vi "Pulse Stretch & Delay.vi"(1 "Delay (sec)":dbl, 2 "In":bool, 4 "Width (sec)":dbl=0.01) -> (5 "Out":bool)   [LabVIEW 2013]
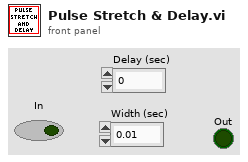
[diagram p1: front panel]
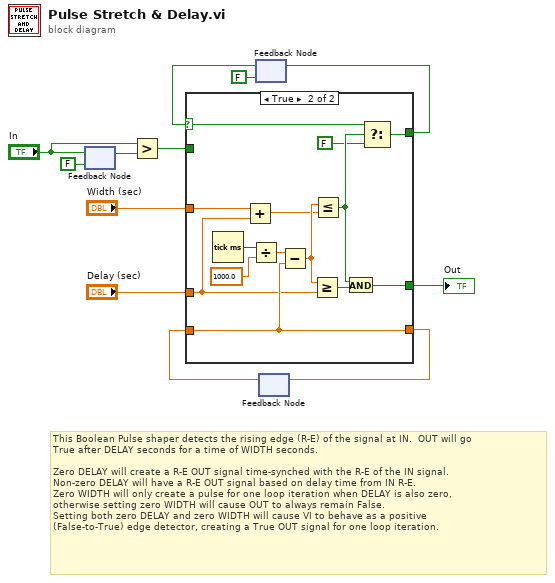
[diagram p0: block diagram]
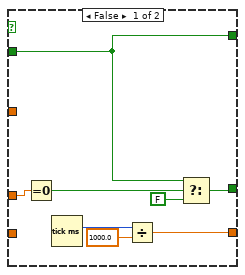
[diagram p2: hidden frame]
diagram:
  # "This Boolean Pulse shaper detects the rising edge (R-E) of the signal at IN.  OUT will go\nTrue after DELAY seconds for a time of WIDTH seconds. \n\nZero DELAY will create a R-E OUT signal time-synched with the R-E of the IN signal.\nNon-zero DELAY will have a R-E OUT signal based on delay time from IN R-E.\nZero WIDTH will only create a pulse for one loop iteration when DELAY is also zero,\notherwise setting zero WIDTH will cause OUT to always remain False.\nSetting both zero DELAY and zero WIDTH will cause VI to behave as a positive\n(False-to-True) edge detector, creating a True OUT signal for one loop iteration."
  n1 = feedback #1(FALSE ("input")) -> (w11:bool)
  n2 = feedback-in #1("In") -> ()
  n3 = Greater?(x="In", y=w11) -> (0:w2:bool)
  n4 = feedback #2(FALSE) -> (w6:bool)
  n5 = feedback #3() -> (w8:dbl)  [unwired: 1 in]
  n6 = case shown="True" w6 {
    selector: w6 -> [_ w27]
    tunnel: [w13 w31] -> w9
    tunnel: w8 -> [_ w31]
    tunnel: [w19 w34] -> w7
    tunnel: w2 -> [w19 _]
    tunnel: [w18 w32] -> w1
    tunnel: "Delay (sec)" -> [w20 w25]
    tunnel: "Width (sec)" -> [_ w24]
    frame False {
      n7 = Equal To 0?(x=w20) -> (x = 0?=w16:bool)
      n8 = Tick Count (ms)() -> (millisecond timer value=w15:u32)
      n9 = Divide(x=w15, y=1000.0) -> (x/y=w13:dbl)
      n10 = Select(t=w19, s=w16, f=FALSE) -> (s? t:f=w18:bool)
    }
    frame True {
      n11 = Tick Count (ms)() -> (millisecond timer value=w22:u32)
      n12 = Add(x=w24, y=w25) -> (x+y=w29:dbl)
      n13 = Divide(x=w22, y=1000.0) -> (x/y=w23:dbl)
      n14 = Subtract(x=w23, y=w31) -> (x-y=w30:dbl)
      n15 = Greater Or Equal?(x=w30, y=w25) -> (x >= y?=w33:bool)
      n16 = Less Or Equal?(x=w30, y=w29) -> (x <= y?=w28:bool)
      n17 = And(x=w28, y=w33) -> (x .and. y?=w32:bool)
      n18 = Select(t=w27, s=w28, f=FALSE) -> (s? t:f=w34:bool)
    }
  }
  "Out" <- w1
  n19 = feedback-in #2(w7) -> ()
  n20 = feedback-in #3(w9) -> ()
